vi "test Add-Find-Remove.vi"(8 "error in":errorcluster, 11 "TestCase in":refnum<class "Scripting.lvclass">) -> (0 "error out":errorcluster, 3 "TestCase out":refnum<class "Scripting.lvclass">)   [LabVIEW 2020, in "Scripting.lvclass"]
uses:
  Scripting.lvclass
  C:/dev/git/niveristand-custom-device-testing-tools/VeriStandScriptingTestCase/VeriStandScriptingTestCase.lvclass
  niveristand-custom-device-testing-tools/VeriStandScriptingTestCase/VeriStandScriptingTestCase.lvclass/VeriStandScriptingTestCase.ctl
  niveristand-custom-device-testing-tools/VeriStandScriptingTestCase/Read Target.vi
  NationalInstruments.VeriStand.SystemDefinitionAPI
  <vilib>/addons/_JKI Toolkits/VI Tester/TestCase.llb/TestCase.lvclass
  Scripting/AIM MIL-STD-1553 Scripting.lvlib
  C:/Program Files (x86)/National Instruments/LabVIEW 2020/vi.lib/addons/_JKI Toolkits/VI Tester/TestCase.llb/TestCase.lvclass
  C:/dev/git/niveristand-aim-milStd1553-custom-device/Source/Custom Device Support/Tests/Unit/Scripting/Scripting.lvclass
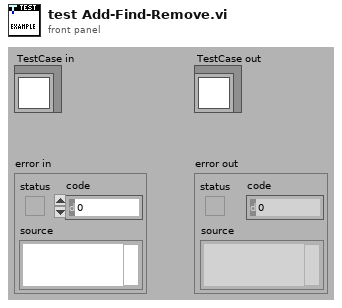
[diagram p1: front panel]
types:
  T1 = typedef "Custom Device API.lvlib/Custom Device Item Ref.ctl" = u64
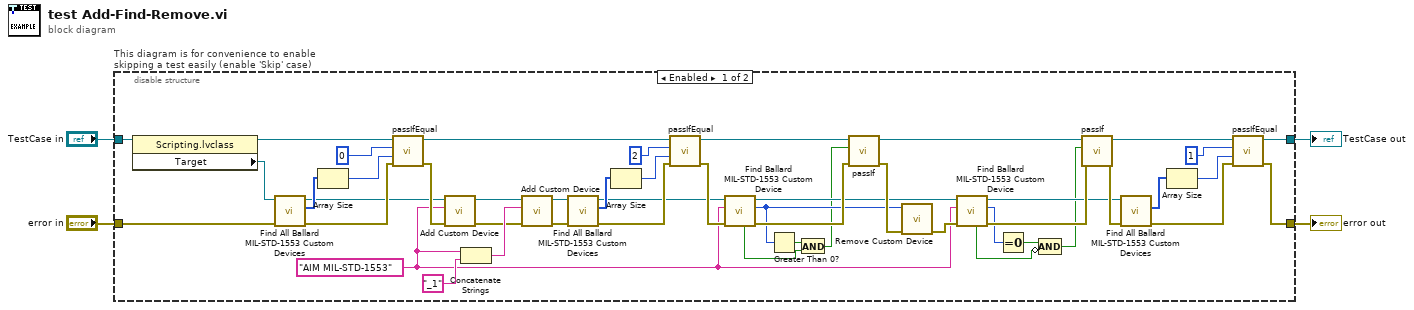
[diagram p0: block diagram]
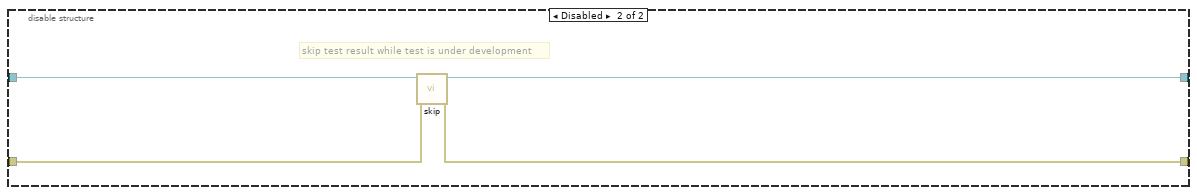
[diagram p2: hidden frame]
diagram:
  n1 = disable-structure "This diagram is for convenience to enable skipping a test easily (enable 'Skip' case)" shown="Enabled" {
    disable-tunnel: "TestCase in" -> [w17 w56]
    disable-tunnel: [w20 w54] -> w1
    disable-tunnel: [w19 w55] -> w3
    disable-tunnel: "error in" -> [w52 w53]
    frame Enabled {
      w30 = "AIM MIL-STD-1553" ("name")
      n2 = property class="Scripting.lvclass"(reference=w17) -> (reference out=w15:refnum<class "Scripting.lvclass">, "Target"=w16:refnum<k24>)  [unwired: 1 in, 1 out]
      n3 = call "Find All Ballard MIL-STD-1553 Custom Devices.vi"("error in"=w52, "target in"=w16) -> ("error out"=w48:errorcluster, "Ballard MIL-STD-1553 custom devices"=w51:T1[], "target out"=w46:refnum<k24>)  [unwired: 7 in]
      n4 = Array Size(array=w51) -> (size(s)=w50:i32)
      n5 = call-dynamic "passIfEqual.vi"("error in (no error)"=w48, "y"=w50, "x"=0 ("size(s)"), "TestCase in"=w15) -> ("error out"=w47:errorcluster, "TestCase out"=w14:refnum<class "Scripting.lvclass">)  [unwired: 6 in]
      n6 = call "Add Custom Device.vi"("error in"=w47, "name"=w30, "target in"=w46) -> ("error out"=w13:errorcluster, "target out"=w44:refnum<k24>)  [unwired: 6 in, 1 out]
      n7 = Concatenate Strings(w30, "_1" ("string")) -> (w43:string)
      n8 = call "Add Custom Device.vi"("error in"=w13, "name"=w43, "target in"=w44) -> ("error out"=w42:errorcluster, "target out"=w41:refnum<k24>)  [unwired: 6 in, 1 out]
      n9 = call "Find All Ballard MIL-STD-1553 Custom Devices.vi"("error in"=w42, "target in"=w41) -> ("error out"=w37:errorcluster, "Ballard MIL-STD-1553 custom devices"=w38:T1[], "target out"=w35:refnum<k24>)  [unwired: 7 in]
      n10 = Array Size(array=w38) -> (size(s)=w39:i32)
      n11 = call-dynamic "passIfEqual.vi"("error in (no error)"=w37, "y"=w39, "x"=2 ("size(s)"), "TestCase in"=w14) -> ("error out"=w36:errorcluster, "TestCase out"=w34:refnum<class "Scripting.lvclass">)  [unwired: 6 in]
      n12 = call "Find Ballard MIL-STD-1553 Custom Device.vi"("error in"=w36, "name"=w30, "target in"=w35) -> ("error out"=w33:errorcluster, "Ballard MIL-STD 1553 custom device"=w11:T1, "target out"=w29:refnum<k24>, "found?"=w8:bool)  [unwired: 5 in]
      n13 = Greater Than 0?(x=w11) -> (x > 0?=w12:bool)
      n14 = And(x=w12, y=w8) -> (x .and. y?=w9:bool)
      n15 = call-dynamic "passIf.vi"("error in (no error)"=w33, "pass"=w9, "TestCase in"=w34) -> ("error out"=w32:errorcluster, "TestCase out"=w28:refnum<class "Scripting.lvclass">)  [unwired: 7 in]
      n16 = call "Remove Custom Device.vi"("error in"=w32, "Ballard MIL-STD 1553 custom device"=w11) -> ("error out"=w31:errorcluster)  [unwired: 9 in]
      n17 = call "Find Ballard MIL-STD-1553 Custom Device.vi"("error in"=w31, "name"=w30, "target in"=w29) -> ("error out"=w27:errorcluster, "Ballard MIL-STD 1553 custom device"=w10:T1, "target out"=w25:refnum<k24>, "found?"=w7:bool)  [unwired: 5 in]
      n18 = Equal To 0?(x=w10) -> (x = 0?=w6:bool)
      n19 = Compound Arithmetic op=AND(w6, invert w7) -> (w5:bool)
      n20 = call-dynamic "passIf.vi"("error in (no error)"=w27, "pass"=w5, "TestCase in"=w28) -> ("error out"=w26:errorcluster, "TestCase out"=w23:refnum<class "Scripting.lvclass">)  [unwired: 7 in]
      n21 = call "Find All Ballard MIL-STD-1553 Custom Devices.vi"("error in"=w26, "target in"=w25) -> ("error out"=w22:errorcluster, "Ballard MIL-STD-1553 custom devices"=w21:T1[])  [unwired: 7 in, 1 out]
      n22 = Array Size(array=w21) -> (size(s)=w18:i32)
      n23 = call-dynamic "passIfEqual.vi"("error in (no error)"=w22, "y"=w18, "x"=1 ("size(s)"), "TestCase in"=w23) -> ("error out"=w19:errorcluster, "TestCase out"=w20:refnum<class "Scripting.lvclass">)  [unwired: 6 in]
    }
    frame Disabled {
      # "skip test result while test is under development"
      n24 = call <vilib>:"skip.vi"("error in (no error)"=w53, "TestCase in"=w56) -> ("error out"=w55:errorcluster, "TestCase out"=w54:refnum<class "Scripting.lvclass">)  [unwired: 8 in]
    }
  }
  "error out" <- w3
  "TestCase out" <- w1
